vi "Prioritizer.vi"(7 "Zone":i32, 9 "Tamper Switches":bool[](array[boolean]), 10 "Bypass Switches":bool[](array[boolean]), 11 "Alarm Switches":bool[](array[boolean])) -> (2 "Zone Status Data":string[](array[string]), 3 "Zone Condition":T1)   [LabVIEW 2016]
doc: "This VI Establishes priority among the alerts received after clicking a switch."
uses:
  Controls/Zones Condition.ctl
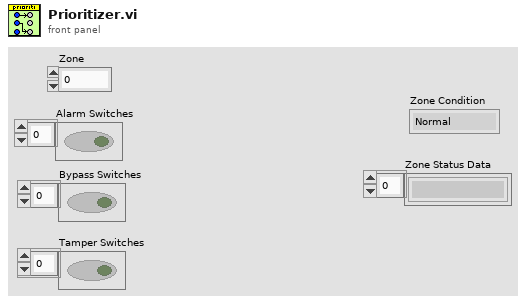
[diagram p1: front panel]
types:
  T1 = typedef "Zones Condition.ctl" = enum16{"Normal", "Bypass", "Tamper", "Alarm"}
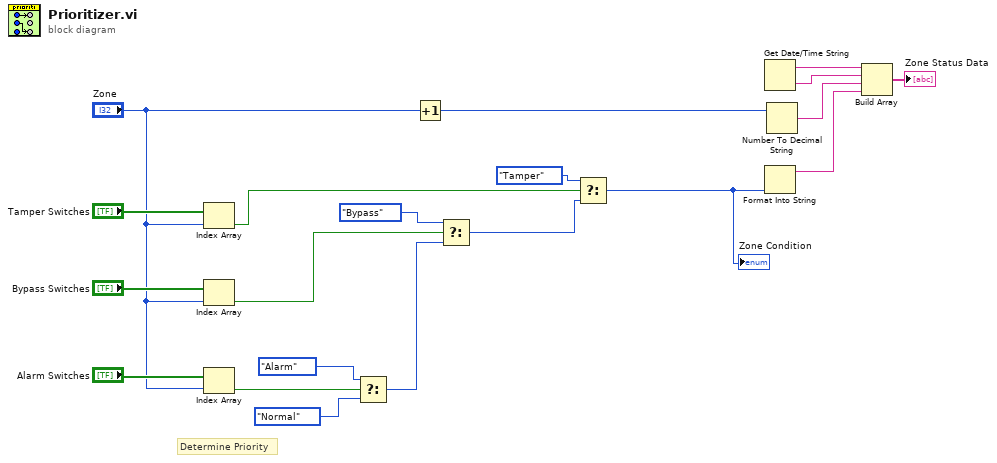
[diagram p0: block diagram]
diagram:
  # "Determine Priority"
  n1 = Index Array(array="Tamper Switches", index="Zone") -> (element=w10:bool)
  n2 = Index Array(array="Bypass Switches", index="Zone") -> (element=w19:bool)
  n3 = Index Array(array="Alarm Switches", index="Zone") -> (element=w14:bool)
  n4 = Select(t=Zones_Condition."Alarm" ("Enum"), s=w14, f=Zones_Condition."Normal" ("Enum")) -> (s? t:f=w13:T1)
  n5 = Increment(x="Zone") -> (x+1=w5:i32)
  n6 = Select(t=Zones_Condition."Bypass", s=w19, f=w13) -> (s? t:f=w9:T1)
  n7 = Select(t=Zones_Condition."Tamper" ("Enum"), s=w10, f=w9) -> (s? t:f=w4:T1)
  "Zone Condition" <- w4
  n8 = Get Date/Time String() -> (date string=w7:string, time string=w6:string)  [unwired: 3 in]
  n9 = Format Into String(w4) -> (resulting string=w2:string)  [unwired: 3 in, 1 out]
  n10 = Number To Decimal String(number=w5) -> (decimal integer string=w3:string)  [unwired: 1 in]
  n11 = Build Array(w7, w6, w3, w2) -> (→"Zone Status Data":string[])
